vi "Handle setConfiguration.vi"(8 "error in (no error)":errorcluster, 10 "setConfiguration":variant, 11 "Instrument.Framework-Template in":refnum<class "Instrument.Framework-Template.lvclass">) -> (0 "error out":errorcluster, 3 "Instrument.Framework-Template out":refnum<class "Instrument.Framework-Template.lvclass">)   [LabVIEW 2019, in "Instrument.Framework-Template.lvclass"]
uses:
  Instrument.Framework-Template.lvclass
  Instrument.Framework-Template.lvclass/Instrument.Framework-Template.ctl
  027c7e6d-2801-4a42-a61c-edfdd76072f6.vi
  027c7e6d-2801-4a42-a61c-edfdd76072f6.vi/de1678d2-7d78-4096-bd73-3b55d853a3c9.vi
  027c7e6d-2801-4a42-a61c-edfdd76072f6.vi/771f1a36-3473-449b-919c-ee613fdfa951.vi
  <vilib>/Utility/Data Type/Get Type Information.vi
  <vilib>/JDP Science/JSONtext/JSON text to Variant.vi
  <vilib>/JDP Science/JSONtext/LVClass Serializer/JSONtext LVClass Serializer.lvclass
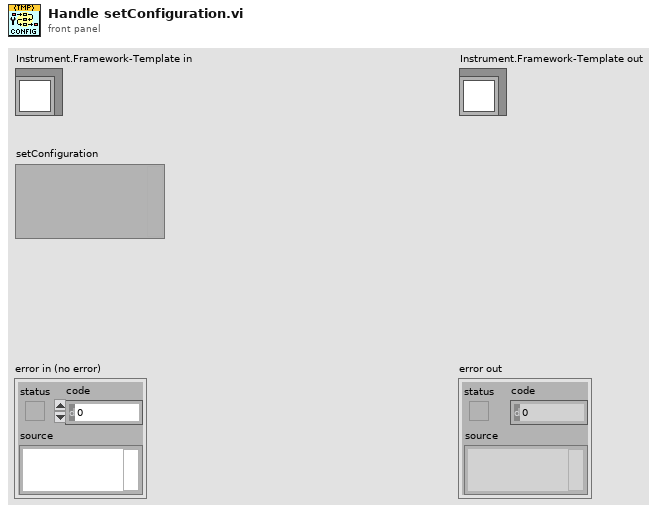
[diagram p1: front panel]
types:
  T1 = typedef "Instrument.Framework-Template.lvclass/Instrument.Framework-Template.Configuration--Cluster.ctl" = cluster{"Example Setting 1":dbl, "Example Setting 2":dbl, "Example Setting 3":string}
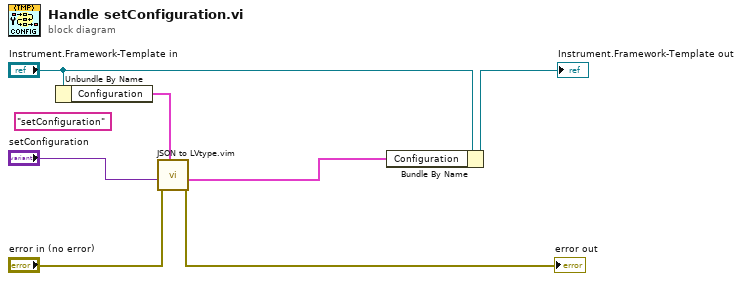
[diagram p0: block diagram]
diagram:
  (unwired) "setConfiguration" ("Command")
  n1 = Unbundle By Name("Instrument.Framework-Template in") -> ("Configuration"=w5:T1)
  n2 = call "JSON to LVtype.vim"("type"=w5, "error in (no error)"="error in (no error)", "JSON Data in"="setConfiguration") -> ("error out"=→"error out":errorcluster, "Data out"=w4:T1)  [unwired: 7 in]
  n3 = Bundle By Name(cluster="Instrument.Framework-Template in", "Configuration"=w4) -> (→"Instrument.Framework-Template out":refnum<class "Instrument.Framework-Template.lvclass">)
